vi "Cluster to Table.vi"(7 "Anything":variant, 11 "Error In":errorcluster) -> (8 "Rows":T1[](array[typedef]), 15 "Error Out":errorcluster)   [LabVIEW 2015, in "KPropertyTable.xctl"]
uses:
  RowData.ctl
  DataType.ctl
  KPropertyTable.xctl
  <vilib>/Utility/Data Type/NI_Data Type.lvlib
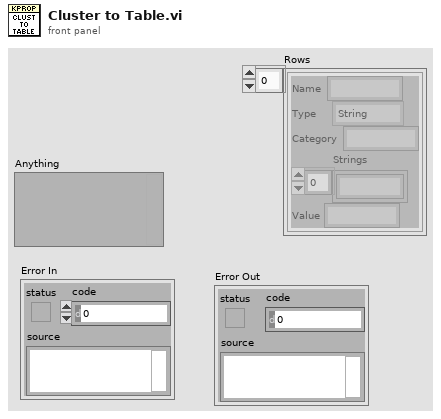
[diagram p1: front panel]
types:
  T1 = typedef "KPropertyTable.xctl/RowData.ctl" = cluster{"Name":string, "Type":T2, "Category":string, "Strings":string[], "Value":string}
  T2 = typedef "KPropertyTable.xctl/DataType.ctl" = enum16{"String", "Enum", "Int", "Double", "Boolean", "Ring", "Formula"}
  T3 = cluster{"Variant":variant, "Name":string, "Cat":string}
  T4 = typedef "NI_Data Type.lvlib/Data Type.ctl" = enum8{"Invalid Type", "Void", "I8", "I16", "I32", "I64", "U8", "U16", "U32", "U64", "Single Float", "Double Float", "Extended Float", "Single Complex", "Double Complex", "Extended Complex", "Enum U8", "Enum U16", "Enum U32", "Enum U64", "Single Float With Unit", "Double Float With Unit", "Extended Float With Unit", "Single Complex with Unit", "Double Complex with Unit", "Extended Complex with Unit", "Boolean", "String", "Path", "Picture", "Tag", "Array", "Cluster", "Variant", "LV Variant", "Waveform", "Timestamp", "Digital Waveform", "Digital Data", "ExpressData", "Refnum", "External Data", "VI", "Poly VI", "LabVIEW Class Instance", "Fixed Point"}
  T5 = cluster{"Variant":variant, string, "Name":string}
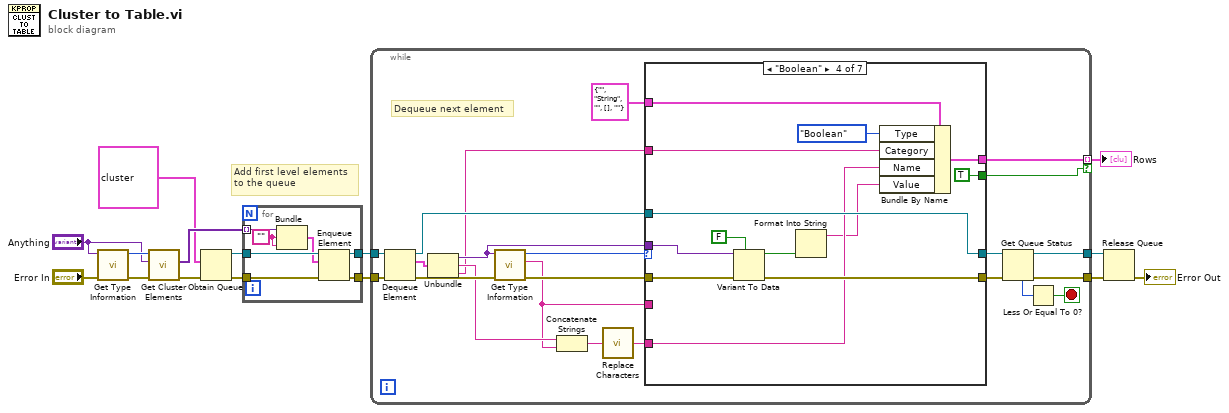
[diagram p0: block diagram]
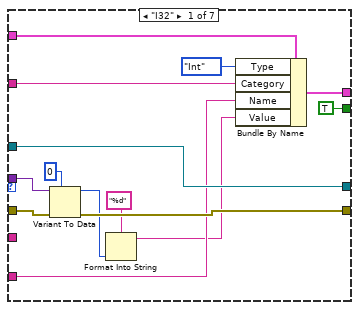
[diagram p2: hidden frame]
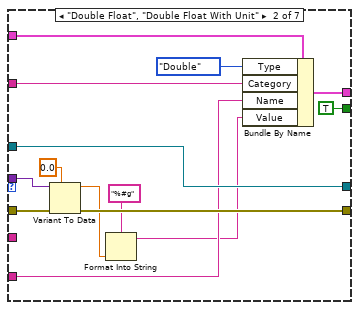
[diagram p3: hidden frame]
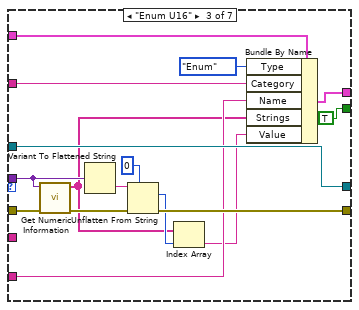
[diagram p4: hidden frame]
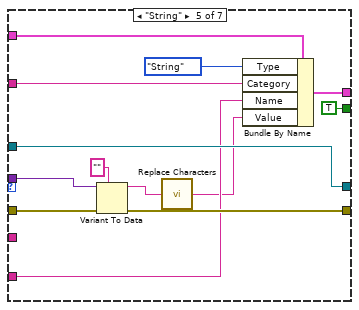
[diagram p5: hidden frame]
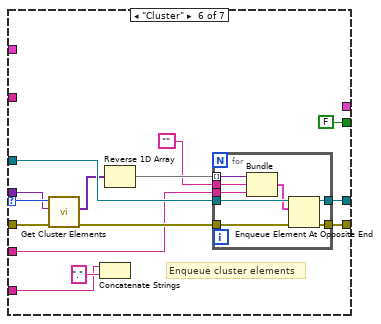
[diagram p6: hidden frame]
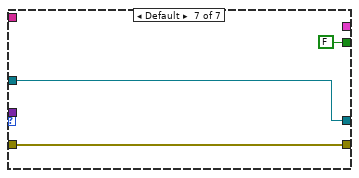
[diagram p7: hidden frame]
diagram:
  # "Add first level elements\nto the queue"
  n1 = call <vilib>:"Get Type Information.vi"("error in (no error)"="Error In", "Variant"="Anything") -> ("error out"=w10:errorcluster, "Type"=w15:T4)  [unwired: 5 in, 3 out]
  n2 = call "Get Cluster Elements.vi"("Error In"=w10, "Cluster"="Anything", "Type Enum (Cluster)"=w15) -> ("Error Out"=w13:errorcluster, "Cluster Elements"=w12:variant[])  [unwired: 7 in]
  n3 = Obtain Queue(element data type=T3 {"Variant"=variant, "Name"="", "Cat"=""}, error in (no error)=w13) -> (queue out=w2:refnum<queue>, error out=w3:errorcluster)  [unwired: 3 in, 1 out]
  n4 = for {
    tunnel: w2 -> [w22]
    tunnel: w3 -> [w21]
    tunnel: [w20] -> w4
    tunnel: [w19] -> w5
    tunnel: w12 -> [w17] mode=indexing
    w16 = ""
    n5 = Bundle("Variant"=w17, w16, w16) -> (w18:cluster{"Variant":variant, string, string})  [unwired: 1 in]
    n6 = Enqueue Element(queue=w22, element=w18, error in (no error)=w21) -> (queue out=w19:refnum<queue>, error out=w20:errorcluster)  [unwired: 1 in, 1 out]
  }
  n7 = while {
    tunnel: w4 -> [w44]
    tunnel: [w41] -> w6
    tunnel: w5 -> [w42]
    tunnel: [w38] -> w7
    tunnel: [w26] -> w1 mode=indexing if=w25
    stop <- w39 stop-if-true
    # "Dequeue next element"
    n8 = Dequeue Element(queue=w42, error in (no error)=w44) -> (queue out=w35:refnum<queue>, element=w33:T3, error out=w43:errorcluster)  [unwired: 1 in, 1 out]
    n9 = Unbundle(w33) -> ("Variant"=w32:variant, "Name"=w31:string, "Cat"=w24:string)
    n10 = call <vilib>:"Get Type Information.vi"("error in (no error)"=w43, "Variant"=w32) -> ("error out"=w30:errorcluster, "Name"=w23:string, "Type"=w37:T4)  [unwired: 5 in, 2 out]
    n11 = Concatenate Strings(w31, w23) -> (w29:string)
    n12 = call "Replace Characters.vi"("String In"=w29) -> ("String Out"=w28:string)  [unwired: 1 in]
    n13 = case shown="\"Boolean\"" w37 {
      selector: w37 -> [_ _ _ _ _ w122 _]
      tunnel: [w58 w72 w88 w101 w114 w126 w139] -> w36
      tunnel: w35 -> [w58 w72 w88 w101 w114 w127 w139]
      tunnel: [w54 w68 w83 w100 w111 w128 w138] -> w34
      tunnel: w30 -> [w57 w71 w87 w97 w113 w124 w138]
      tunnel: w28 -> [w49 w63 w78 w94 w106 w118 _]
      tunnel: w32 -> [w56 w70 w86 w98 w110 w121 _]
      tunnel: T1 {"Name"="", "Type"=enum."String", "Category"="", "Strings"=[], "Value"=""} ("Row") -> [w51 w65 w80 w96 w108 _ _]
      tunnel: [w47 w61 w75 w91 w104 _ _] -> w26
      tunnel: [TRUE TRUE TRUE TRUE TRUE FALSE FALSE] -> w25
      tunnel: w24 -> [w45 w59 w73 w89 w102 _ _]
      tunnel: w23 -> [_ _ _ _ _ w116 _]
      frame "I32" {
        n14 = Variant To Data(error in=w57, type=0, Variant=w56) -> (data=w53:i32, error out=w54:errorcluster)
        n15 = Format Into String(format string="%d", w53) -> (resulting string=w48:string)  [unwired: 2 in, 1 out]
        n16 = Bundle By Name(cluster=w51, "Type"=DataType."Int", "Category"=w45, "Name"=w49, "Value"=w48) -> (w47:T1)
      }
      frame "Double Float", "Double Float With Unit" {
        n17 = Variant To Data(error in=w71, type=0.0, Variant=w70) -> (data=w67:dbl, error out=w68:errorcluster)
        n18 = Format Into String(format string="%#g", w67) -> (resulting string=w62:string)  [unwired: 2 in, 1 out]
        n19 = Bundle By Name(cluster=w65, "Type"=DataType."Double", "Category"=w59, "Name"=w63, "Value"=w62) -> (w61:T1)
      }
      frame "Enum U16" {
        n20 = call <vilib>:"Get Numeric Information.vi"("error in (no error)"=w87, "Variant"=w86) -> ("error out"=w84:errorcluster, "Enum Names"=w77:string[])  [unwired: 6 in, 2 out]
        n21 = Variant To Flattened String(Variant=w86) -> (data string=w85:string)  [unwired: 1 out]
        n22 = Unflatten From String(type=u8 0, binary string=w85, error in (no error)=w84) -> (value=w82:u8, error out=w83:errorcluster)  [unwired: 2 in, 1 out]
        n23 = Index Array(array=w77, index=w82) -> (element=w76:string)
        n24 = Bundle By Name(cluster=w80, "Type"=DataType."Enum", "Category"=w73, "Name"=w78, "Strings"=w77, "Value"=w76) -> (w75:T1)
      }
      frame "Boolean" {
        n25 = Variant To Data(error in=w97, type=FALSE, Variant=w98) -> (data=w93:bool, error out=w100:errorcluster)
        n26 = Format Into String(w93) -> (resulting string=w92:string)  [unwired: 3 in, 1 out]
        n27 = Bundle By Name(cluster=w96, "Type"=DataType."Boolean", "Category"=w89, "Name"=w94, "Value"=w92) -> (w91:T1)
      }
      frame "String" {
        n28 = Variant To Data(error in=w113, type="", Variant=w110) -> (data=w112:string, error out=w111:errorcluster)
        n29 = call "Replace Characters.vi"("String In"=w112) -> ("String Out"=w105:string)  [unwired: 1 in]
        n30 = Bundle By Name(cluster=w108, "Type"=DataType."String", "Category"=w102, "Name"=w106, "Value"=w105) -> (w104:T1)
      }
      frame "Cluster" {
        # "Enqueue cluster elements"
        n31 = call "Get Cluster Elements.vi"("Error In"=w124, "Cluster"=w121, "Type Enum (Cluster)"=w122) -> ("Error Out"=w123:errorcluster, "Cluster Elements"=w120:variant[])  [unwired: 7 in]
        n32 = Concatenate Strings(w118, "." ("string")) -> ()  [unwired: 1 out]
        n33 = Reverse 1D Array(array=w120) -> (reversed array=w125:variant[])
        n34 = for {
          tunnel: w127 -> [w136]
          tunnel: w123 -> [w135]
          tunnel: [w134] -> w128
          tunnel: [w133] -> w126
          tunnel: w125 -> [w131] mode=indexing
          tunnel: "" -> [w130]
          tunnel: w116 -> [w129]
          n35 = Bundle("Variant"=w131, w130, "Name"=w129) -> (w132:T5)  [unwired: 1 in]
          n36 = Enqueue Element At Opposite End(queue=w136, element=w132, error in (no error)=w135) -> (queue out=w133:refnum<queue>, error out=w134:errorcluster)  [unwired: 1 in, 1 out]
        }
      }
      frame Default {
      }
    }
    n37 = Get Queue Status(queue=w36, error in (no error)=w34) -> (queue out=w38:refnum<queue>, error out=w41:errorcluster, # elements in queue=w40:i32)  [unwired: 1 in, 5 out]
    n38 = Less Or Equal To 0?(x=w40) -> (x <= 0?=w39:bool)
  }
  "Rows" <- w1
  n39 = Release Queue(queue=w7, error in (no error)=w6) -> (error out=→"Error Out":errorcluster)  [unwired: 1 in, 2 out]
